vi "loadSTLtest.vi"() -> ()   [LabVIEW 2022 SP3]
uses:
  coordSys.ctl
  <vilib>/picture/3D Picture Control/Object/Create Object (name).vi
  <vilib>/picture/3D Picture Control/Object/Add Object (reference).vi
  <vilib>/picture/3D Picture Control/NI_3D Picture Control.lvlib
panel:
  in  "diagram":i32=1
  out "stlObjectOut":refnum<vi>
  out "error out":errorcluster
  in  "Job Directory":path=path "/Users/tlawton/LocalDataCache/Projects/19904"
  in  "error in (no error)":errorcluster
  in  "modelColours":u32[](array[colorbox])
  in  "STLs":cluster{"coordSys":T1, "WD":dbl, "STL":string}[](array[cluster])=[{"coordSys"=enum."Model", "WD"=0.0, "STL"="STLs"}]
  in  "Alpha":dbl
  out "3D Picture":refnum<vi>(3d-picture)
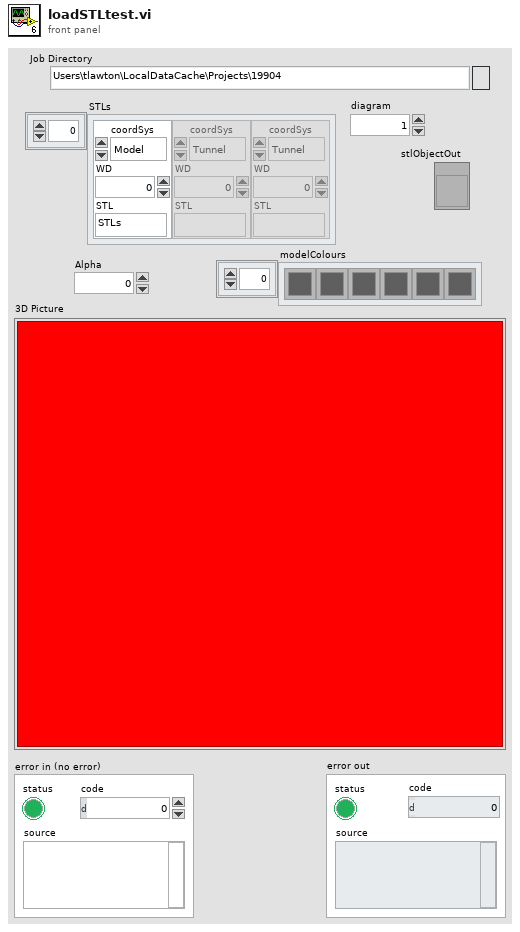
[diagram p1: front panel]
types:
  T1 = typedef "coordSys.ctl" = enum16{"Tunnel", "Model"}
  T2 = enum16{"Inherit Value", "Points", "Wireframe", "Polygons"}
  T3 = enum16{"Inherit Value", "No Culling", "Cull Back Face", "Cull Front Face", "Cull Both Faces"}
  T4 = enum16{"Inherit Value", "Counterclockwise", "Clockwise"}
  T5 = typedef "Triangle.ctl" = cluster{"V0":sgl[], "V1":sgl[], "V2":sgl[], "E0":sgl[], "E1":sgl[], "E2":sgl[], "n^":sgl[], "nE0^":sgl[], "nE1^":sgl[], "nE2^":sgl[]}
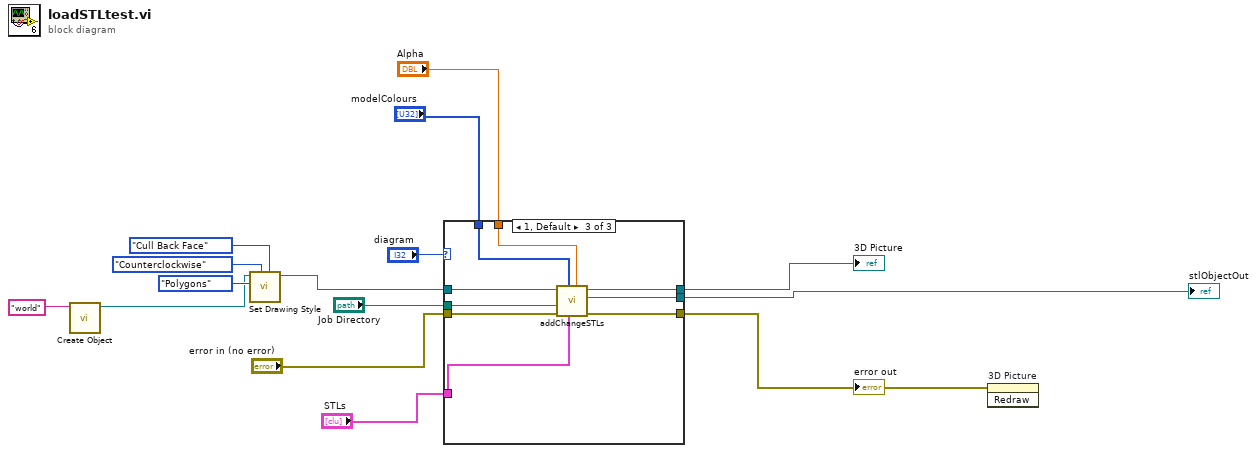
[diagram p0: block diagram]
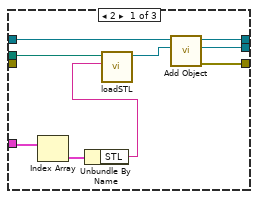
[diagram p2: hidden frame]
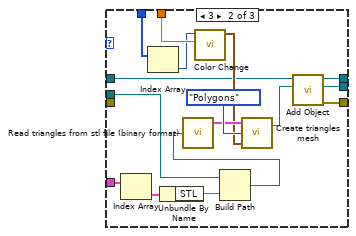
[diagram p3: hidden frame]
diagram:
  n1 = call-poly <vilib>:"Create Object.vi"("Name"="world") -> ("Scene:New Object"=w5:refnum<vi>)  [unwired: 9 in, 1 out]
  n2 = call <vilib>:"Set Drawing Style.vi"("Face Culling Mode"=T3."Cull Back Face", "Frontface Mode"=T4."Counterclockwise", "Mode"=T2."Polygons", "Scene Object In"=w5) -> ("Scene Object Out"=w3:refnum<vi>)  [unwired: 6 in, 1 out]
  n3 = case shown="1, Default" "diagram" {
    tunnel: w3 -> [w22 w33 w49]
    tunnel: [w23 w32 w48] -> w2
    tunnel: "Alpha" -> [_ w37 w47]
    tunnel: "STLs" -> [w21 w29 w46]
    tunnel: "modelColours" -> [_ w38 w45]
    tunnel: "error in (no error)" -> [_ _ w44]
    tunnel: "Job Directory" -> [w18 w26 w43]
    tunnel: [w17 w31 w42] -> w1
    tunnel: [w16 w30 w41] -> w10
    frame 2 {
      n4 = Index Array(array=w21) -> (element=w20:cluster{"coordSys":T1, "WD":dbl, "STL":string})  [unwired: 1 in]
      n5 = Unbundle By Name(w20) -> ("STL"=w19:string)
      n6 = call "loadSTL.vi"("STLname"=w19, "Job Directory"=w18) -> ("SceneObject out"=w24:refnum<vi>)  [unwired: 8 in, 1 out]
      n7 = call-poly <vilib>:"Add Object.vi"("New Object In"=w24, "Scene Object In"=w22) -> ("error out"=w17:errorcluster, "New Object Out"=w16:refnum<vi>, "Scene Object Out"=w23:refnum<vi>)  [unwired: 7 in]
    }
    frame 3 {
      n8 = Index Array(array=w29) -> (element=w28:cluster{"coordSys":T1, "WD":dbl, "STL":string})  [unwired: 1 in]
      n9 = Index Array(array=w38) -> (element=w36:u32)  [unwired: 1 in]
      n10 = Unbundle By Name(w28) -> ("STL"=w27:string)
      n11 = call <vilib>:"Color Change.vi"("Alpha"=w37, "Color"=w36) -> ("RGBA"=w35:cluster{"R":sgl, "G":sgl, "B":sgl, "A":sgl})  [unwired: 9 in]
      n12 = Build Path(base path=w26, name or relative path=w27) -> (appended path=w25:path)
      n13 = call "Read triangles from stl file (binary format).vi"("STL file path"=w25) -> ("Triangles array"=w39:T5[])  [unwired: 2 out]
      n14 = call "Create triangles mesh.vi"("Colour"=w35, "Render mode"=T2."Polygons", "Triangles array"=w39) -> ("Triangle mesh out"=w34:refnum<vi>)  [unwired: 1 out]
      n15 = call-poly <vilib>:"Add Object.vi"("New Object In"=w34, "Scene Object In"=w33) -> ("error out"=w31:errorcluster, "New Object Out"=w30:refnum<vi>, "Scene Object Out"=w32:refnum<vi>)  [unwired: 7 in]
    }
    frame 1, Default {
      n16 = call "addChangeSTLs.vi"("Alpha"=w47, "STLs"=w46, "modelColours"=w45, "error in (no error)"=w44, "Job Directory"=w43, "parentObjectIn"=w49) -> ("error out"=w42:errorcluster, "stlObjectOut"=w41:refnum<vi>, "parentObjectOut"=w48:refnum<vi>)  [unwired: 3 in]
    }
  }
  "3D Picture" <- w2
  "error out" <- w1
  "stlObjectOut" <- w10
  n17 = invoke on="3D Picture" class="SceneGraphDisp (strict)" method="Redraw"(error in=w1) -> ()  [unwired: 2 in, 3 out]
